vi "Teleop.vi"(0 "Call Context":T10) -> (6 "SubState 3":T4, 8 "SubState 4":T4, 9 "SubState 5":T9, 11 "Loop 3 Data":T5, 13 "Loop 4 Data":T3, 14 "SubState 0":T4=enum."driver control", 15 "Loop 1 Data":T7, 16 "Loop 0 Data":T8, 17 "SubState 1":T4, 18 "Loop 2 Data":T6, 19 "SubState 2":T4)   [LabVIEW 2013]
uses:
  typedefs/subStates.ctl
  <vilib>/Rock Robotics/WPI/DriverStation/WPI_DriverStationDerivedRobotMode.ctl
  typedefs/singleUseSubstate.ctl
  typedefs/Loop Datatypes/Loop 0 Datatype.ctl
  typedefs/Loop Datatypes/Loop 1 Datatype.ctl
  typedefs/Loop Datatypes/Loop 2 Datatype.ctl
  typedefs/Loop Datatypes/Loop 3 Datatype.ctl
  typedefs/Loop Datatypes/Loop 4 Datatype.ctl
  <vilib>/Rock Robotics/WPI/Joystick/WPI_JoystickDevRef.ctl
  <vilib>/Rock Robotics/WPI/Joystick/WPI_JoystickDeviceEnum.ctl
  typedefs/fg_typedef.ctl
  <vilib>/Rock Robotics/WPI/Joystick/WPI_JoystickGetSetRefNum.vi
panel:
  out "Drive to DC":bool
  out "JS2 Button 9":bool
  out "JS3":T1
  out "JS1":T1
  out "JS2":T1
  out "Exit Value":i32=-1
  # "Loop Data and Substates"
  # "Drive Loop"
  # "Shooter Pneumatics Loop"
  # "Pickup/Passing Belts Loop"
  # "Pickup Arm Loop"
  # "Unassigned Loop"
  # "Shifter Loop"
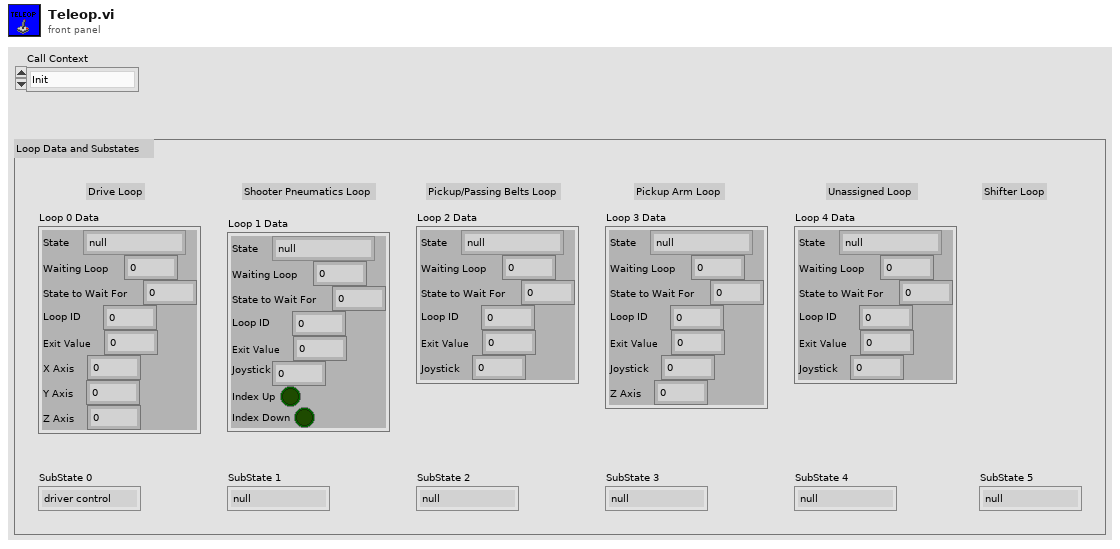
[diagram p1: front panel]
types:
  T1 = typedef "WPI_JoystickDevRef.ctl" = cluster{"Device":T2}
  T2 = typedef "WPI_JoystickDeviceEnum.ctl" = enum16{"USB 1", "USB 2", "USB 3", "USB 4", "Kinect 1", "Kinect 2"}
  T3 = typedef "Loop 4 Datatype.ctl" = cluster{"State":T4, "Waiting Loop":i32, "State to Wait For":i32, "Loop ID":i32, "Exit Value":i32, "Joystick":dbl}
  T4 = typedef "subStates.ctl" = enum16{"null", "wait", "driver control", "auto", "manual override", "hold position", "rotate", "pickup", "pass", "load", "cock", "goto shoot", "shoot", "end"}
  T5 = typedef "Loop 3 Datatype.ctl" = cluster{"State":T4, "Waiting Loop":i32, "State to Wait For":i32, "Loop ID":i32, "Exit Value":i32, "Joystick":dbl, "Z Axis":dbl}
  T6 = typedef "Loop 2 Datatype.ctl" = cluster{"State":T4, "Waiting Loop":i32, "State to Wait For":i32, "Loop ID":i32, "Exit Value":i32, "Joystick":dbl}
  T7 = typedef "Loop 1 Datatype.ctl" = cluster{"State":T4, "Waiting Loop":i32, "State to Wait For":i32, "Loop ID":i32, "Exit Value":i32, "Joystick":dbl, "Index Up":bool, "Index Down":bool}
  T8 = typedef "Loop 0 Datatype.ctl" = cluster{"State":T4, "Waiting Loop":i32, "State to Wait For":i32, "Loop ID":i32, "Exit Value":i32, "X Axis":dbl, "Y Axis":dbl, "Z Axis":dbl}
  T9 = typedef "singleUseSubstate.ctl" = enum16{"null", "wait", "shift high", "shift low"}
  T10 = typedef "WPI_DriverStationDerivedRobotMode.ctl" = enum16{"Init", "Execute", "Stop"}
  T11 = cluster{"axis 1 (x)":dbl, "axis 2 (y)":dbl, "axis 3 (throttle)":dbl, "axis 4":dbl, "axis 5":dbl, "axis 6":dbl}
  T12 = typedef "WPI_JoystickButtonState.ctl" = cluster{"Button 1":bool, "Button 2":bool, "Button 3":bool, "Button 4":bool, "Button 5":bool, "Button 6":bool, "Button 7":bool, "Button 8":bool, "Button 9":bool, "Button 10":bool, "Button 11":bool, "Button 12":bool}
  T13 = typedef "WPI_EncoderDevRef.ctl" = cluster{"DevStatus":errorcluster, "EncoderIndex":T14, "CounterIndex":T15, "DistancePerCount":dbl, "Decoding Type":T16}
  T14 = typedef "FPGA_EncoderIdx.ctl" = enum8{"Enc 0", "Enc 1", "Enc 2", "Enc 3", "Invalid"}
  T15 = typedef "FPGA_CounterCtrSystemIndex.ctl" = enum8{"Ctr 0", "Ctr 1", "Ctr 2", "Ctr 3", "Ctr 4", "Ctr 5", "Ctr 6", "Ctr 7", "Invalid"}
  T16 = typedef "WPI_EncoderType.ctl" = enum16{"1x", "2x", "4x"}
  T17 = typedef "fg_typedef.ctl" = enum16{"Get", "Set"}
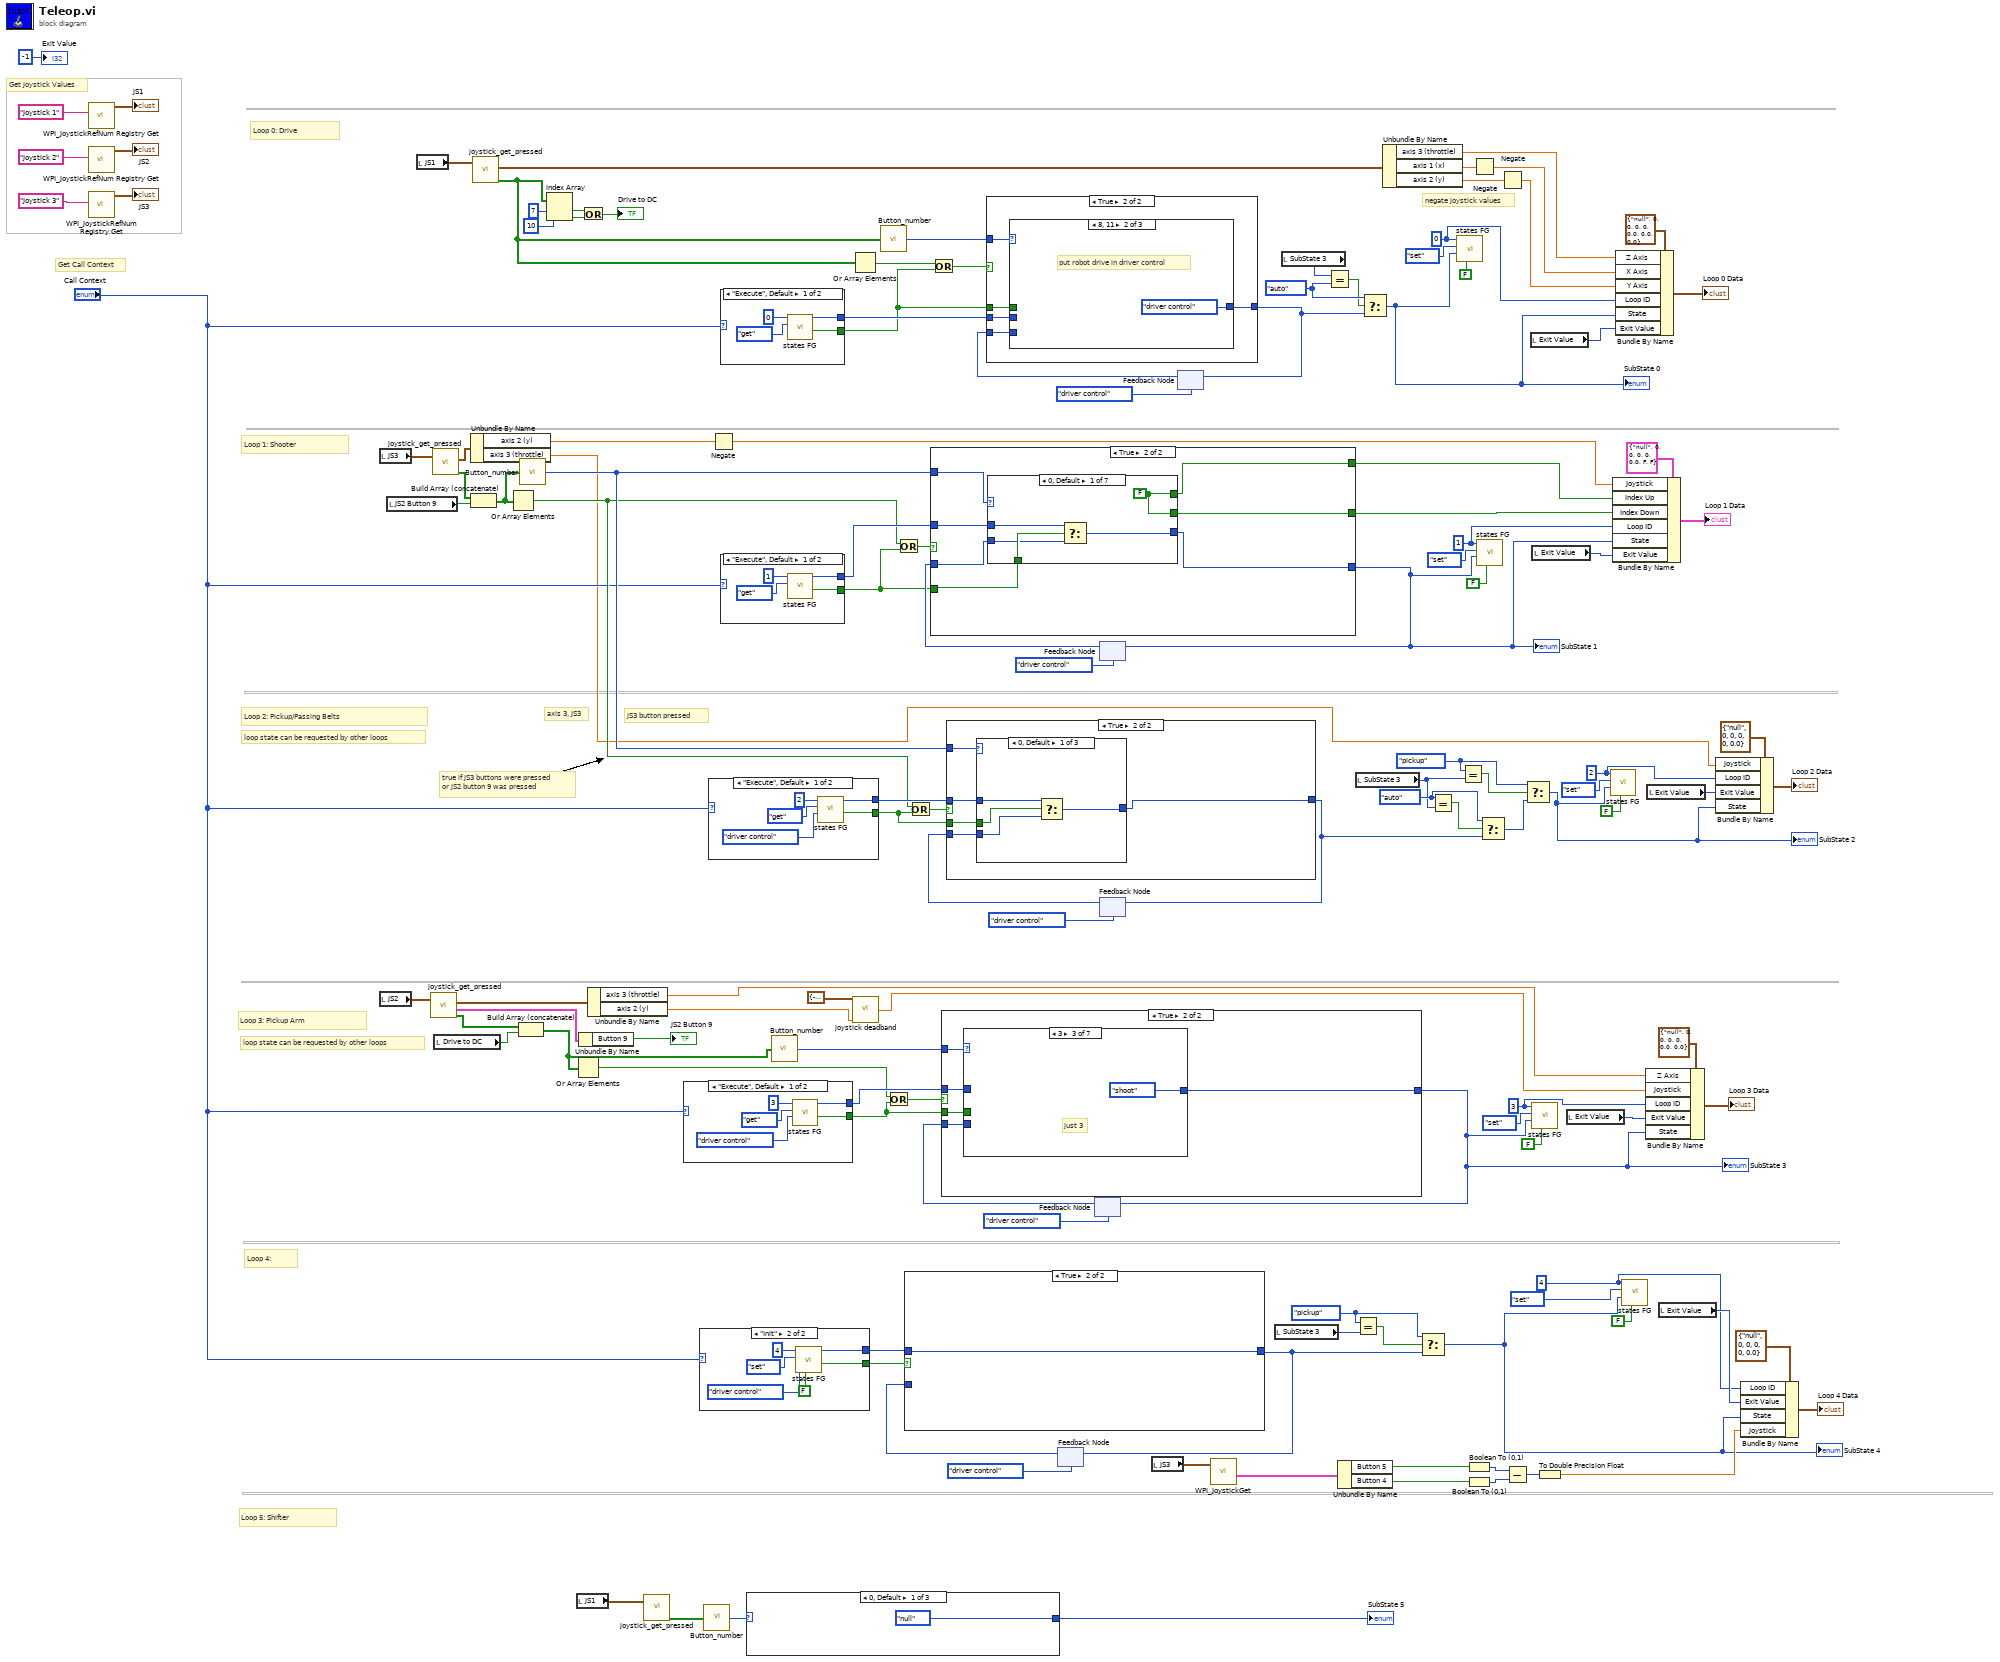
[diagram p0: block diagram]
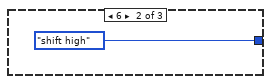
[diagram p2: hidden frame]
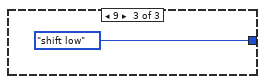
[diagram p3: hidden frame]
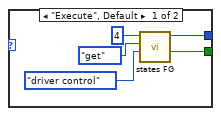
[diagram p5: hidden frame]
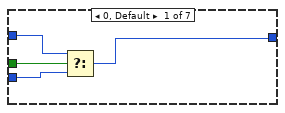
[diagram p7: hidden frame]
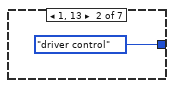
[diagram p8: hidden frame]
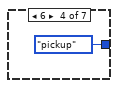
[diagram p9: hidden frame]
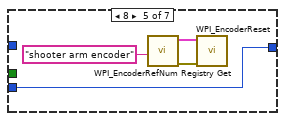
[diagram p10: hidden frame]
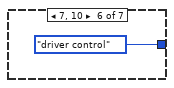
[diagram p11: hidden frame]
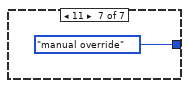
[diagram p12: hidden frame]
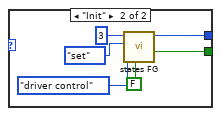
[diagram p13: hidden frame]
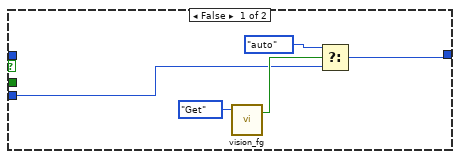
[diagram p14: hidden frame]
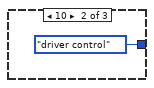
[diagram p15: hidden frame]
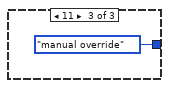
[diagram p16: hidden frame]
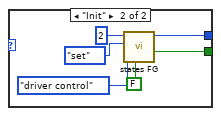
[diagram p17: hidden frame]
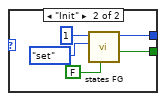
[diagram p18: hidden frame]
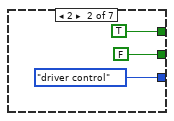
[diagram p20: hidden frame]
diagram:
  w26 = subStates."auto" ("y")
  w29 = subStates."auto" ("x")
  w36 = subStates."pickup" ("x")
  w38 = subStates."pickup" ("x")
  w91 = 4 ("Loop ID")
  w106 = 3 ("Loop ID")
  w107 = 2 ("Loop ID")
  w116 = 1 ("Loop ID")
  w118 = 0 ("Loop ID")
  # "true if JS3 buttons were pressed\nor JS2 button 9 was pressed"
  # "JS3 button pressed"
  # "axis 3, JS3"
  # "negate joystick values"
  # "Get Call Context"
  # "Get Joystick Values"
  # "Loop 4:"
  # "Loop 3: Pickup Arm"
  # "loop state can be requested by other loops"
  # "Loop 5: Shifter"
  # "Loop 2: Pickup/Passing Belts"
  # "Loop 1: Shooter"
  # "Loop 0: Drive"
  # "loop state can be requested by other loops"
  n1 = call <vilib>:"WPI_JoystickRefNum Registry Get.vi"("refnum name"="Joystick 1") -> ("JoystickDevRef"=→"JS1":T1)  [unwired: 9 in, 1 out]
  n2 = call <vilib>:"WPI_JoystickRefNum Registry Get.vi"("refnum name"="Joystick 2") -> ("JoystickDevRef"=→"JS2":T1)  [unwired: 9 in, 1 out]
  n3 = call <vilib>:"WPI_JoystickRefNum Registry Get.vi"("refnum name"="Joystick 3") -> ("JoystickDevRef"=→"JS3":T1)  [unwired: 9 in, 1 out]
  n4 = local read "JS3"() -> (w71:T1)
  n5 = local read "JS2"() -> (w49:T1)
  n6 = local read "JS2 Button 9"() -> (w56:bool)
  n7 = local read "JS1"() -> (w72:T1)
  n8 = call "joystick_get_pressed.vi"("JoystickDevRef 2"=w49) -> ("Axes"=w54:T11, "Buttons"=w8:T12, "Buttons Pressed?"=w52:bool[])  [unwired: 1 in, 1 out]
  n9 = call "joystick_get_pressed.vi"("JoystickDevRef 2"=w71) -> ("Axes"=w70:T11, "Buttons Pressed?"=w32:bool[])  [unwired: 1 in, 2 out]
  n10 = local read "Drive to DC"() -> (w11:bool)
  n11 = Unbundle By Name(w70) -> ("axis 2 (y)"=w79:dbl, "axis 3 (throttle)"=w6:dbl)
  n12 = Build Array (concatenate)(w32, w56) -> (w31:bool[])
  n13 = call "joystick_get_pressed.vi"("JoystickDevRef 2"=w72) -> ("Axes"=w78:T11, "Buttons Pressed?"=w17:bool[])  [unwired: 1 in, 2 out]
  n14 = Or Array Elements(Boolean array=w31) -> (logical OR=w59:bool)
  n15 = Build Array (concatenate)(w52, w11) -> (w5:bool[])
  n16 = call "Button_number.vi"("Button Array"=w31) -> ("Button Pressed"=w61:i32)
  n17 = Index Array(array=w17, index #1=7 ("index"), index #2=10 ("index")) -> (element #1=w14:bool, element #2=w13:bool)
  n18 = Or Array Elements(Boolean array=w5) -> (logical OR=w53:bool)
  n19 = local read "JS1"() -> (w1:T1)
  n20 = Unbundle By Name(w8) -> ("Button 9"=→"JS2 Button 9":bool)
  n21 = Or(x=w14, y=w13) -> (x .or. y?=→"Drive to DC":bool)
  n22 = Unbundle By Name(w54) -> ("axis 3 (throttle)"=w19:dbl, "axis 2 (y)"=w22:dbl)
  n23 = call "joystick_get_pressed.vi"("JoystickDevRef 2"=w1) -> ("Buttons Pressed?"=w3:bool[])  [unwired: 1 in, 3 out]
  n24 = case shown="\"Execute\", Default" "Call Context" {
    tunnel: [w137 w143] -> w50
    tunnel: [w135 w140] -> w104
    frame "Execute", Default {
      n25 = call "states FG.vi"("subState in"=subStates."driver control", "menu (get)"=enum16{"set", "get"}."get", "Loop ID"=3) -> ("exit out"=w137:bool, "subState out"=w135:T4)  [unwired: 5 in, 2 out]
    }
    frame "Init" {
      n26 = call "states FG.vi"("exit in"=FALSE, "subState in"=subStates."driver control", "menu (get)"=enum16{"set", "get"}."set", "Loop ID"=3) -> ("exit out"=w143:bool, "subState out"=w140:T4)  [unwired: 4 in, 2 out]
    }
  }
  n27 = case shown="\"Init\"" "Call Context" {
    tunnel: [w148 w154] -> w46
    tunnel: [w146 w151] -> w93
    frame "Execute", Default {
      n28 = call "states FG.vi"("subState in"=subStates."driver control", "menu (get)"=enum16{"set", "get"}."get", "Loop ID"=4) -> ("exit out"=w148:bool, "subState out"=w146:T4)  [unwired: 5 in, 2 out]
    }
    frame "Init" {
      n29 = call "states FG.vi"("exit in"=FALSE, "subState in"=subStates."driver control", "menu (get)"=enum16{"set", "get"}."set", "Loop ID"=4) -> ("exit out"=w154:bool, "subState out"=w151:T4)  [unwired: 4 in, 2 out]
    }
  }
  n30 = call "Button_number.vi"("Button Array"=w3) -> ("Button Pressed"=w2:i32)
  n31 = case shown="\"Execute\", Default" "Call Context" {
    tunnel: [w159 w165] -> w58
    tunnel: [w157 w162] -> w123
    frame "Execute", Default {
      n32 = call "states FG.vi"("subState in"=subStates."driver control", "menu (get)"=enum16{"set", "get"}."get", "Loop ID"=2) -> ("exit out"=w159:bool, "subState out"=w157:T4)  [unwired: 5 in, 2 out]
    }
    frame "Init" {
      n33 = call "states FG.vi"("exit in"=FALSE, "subState in"=subStates."driver control", "menu (get)"=enum16{"set", "get"}."set", "Loop ID"=2) -> ("exit out"=w165:bool, "subState out"=w162:T4)  [unwired: 4 in, 2 out]
    }
  }
  n34 = Negate(x=w79) -> (-x=w64:dbl)
  n35 = case shown="\"Execute\", Default" "Call Context" {
    tunnel: [w169 w174] -> w68
    tunnel: [w168 w172] -> w121
    frame "Execute", Default {
      n36 = call "states FG.vi"("menu (get)"=enum16{"set", "get"}."get", "Loop ID"=0) -> ("exit out"=w169:bool, "subState out"=w168:T4)  [unwired: 6 in, 2 out]
    }
    frame "Init" {
      n37 = call "states FG.vi"("exit in"=FALSE, "menu (get)"=enum16{"set", "get"}."set", "Loop ID"=0) -> ("exit out"=w174:bool, "subState out"=w172:T4)  [unwired: 5 in, 2 out]
    }
  }
  n38 = case shown="\"Execute\", Default" "Call Context" {
    tunnel: [w178 w183] -> w65
    tunnel: [w177 w181] -> w120
    frame "Execute", Default {
      n39 = call "states FG.vi"("menu (get)"=enum16{"set", "get"}."get", "Loop ID"=1) -> ("exit out"=w178:bool, "subState out"=w177:T4)  [unwired: 6 in, 2 out]
    }
    frame "Init" {
      n40 = call "states FG.vi"("exit in"=FALSE, "menu (get)"=enum16{"set", "get"}."set", "Loop ID"=1) -> ("exit out"=w183:bool, "subState out"=w181:T4)  [unwired: 5 in, 2 out]
    }
  }
  n41 = case shown="0, Default" w2 {
    tunnel: [singleUseSubstate."null" ("Enum") singleUseSubstate."shift high" ("Enum") singleUseSubstate."shift low" ("Enum")] -> w88
    frame 0, Default {
    }
    frame 6 {
    }
    frame 9 {
    }
  }
  "SubState 5" <- w88
  n42 = call "Button_number.vi"("Button Array"=w5) -> ("Button Pressed"=w51:i32)
  n43 = Or Array Elements(Boolean array=w17) -> (logical OR=w69:bool)
  n44 = call "joystick deadband.vi"("Joystick In"=w22, "Deadband Range"=cluster{"Deadband Min":dbl, "Deadband Max":dbl} {"Deadband Min"=-0.05, "Deadband Max"=0.05}) -> ("Joystick Out"=w4:dbl)  [unwired: 4 in]
  n45 = call "Button_number.vi"("Button Array"=w17) -> ("Button Pressed"=w77:i32)
  n46 = Or(x=w53, y=w50) -> (x .or. y?=w55:bool)
  n47 = Or(x=w59, y=w65) -> (x .or. y?=w66:bool)
  n48 = Or(x=w59, y=w58) -> (x .or. y?=w60:bool)
  n49 = Or(x=w69, y=w68) -> (x .or. y?=w67:bool)
  n50 = feedback #1(subStates."driver control" ("Drive SubState")) -> (w96:T4)
  n51 = case shown="True" w46 {
    tunnel: w96 -> [w189 _]
    tunnel: [w189 w190] -> w33
    tunnel: w93 -> [_ w190]
    frame False {
    }
    frame True {
    }
  }
  n52 = feedback-in #1(w33) -> ()
  n53 = feedback #2(subStates."driver control" ("Drive SubState")) -> (w101:T4)
  n54 = case shown="True" w55 {
    tunnel: w101 -> [w191 w192]
    tunnel: [w191 w193] -> w80
    tunnel: w104 -> [_ w194]
    tunnel: w51 -> [_ w196]
    tunnel: w50 -> [_ w195]
    frame False {
    }
    frame True {
      n55 = case shown="3" w196 {
        tunnel: w195 -> [w200 _ _ _ _ _ _]
        tunnel: w192 -> [w199 _ _ _ w204 _ _]
        tunnel: w194 -> [w198 _ _ _ _ _ _]
        tunnel: [w197 subStates."driver control" ("Drive SubState") subStates."shoot" ("Drive SubState") subStates."pickup" ("Drive SubState") w204 subStates."driver control" ("Drive SubState") subStates."manual override" ("Drive SubState")] -> w193
        frame 0, Default {
          n56 = Select(t=w198, s=w200, f=w199) -> (s? t:f=w197:T4)
        }
        frame 1, 13 {
        }
        frame 3 {
          # "just 3"
        }
        frame 6 {
        }
        frame 8 {
          n57 = call <vilib>:"WPI_EncoderRefNum Registry Get.vi"("refnum name"="shooter arm encoder") -> ("error out"=w206:errorcluster, "EncoderDevRef"=w205:T13)  [unwired: 9 in]
          n58 = call <vilib>:"WPI_EncoderReset.vi"("error in (no error)"=w206, "EncoderDevRef"=w205) -> ()  [unwired: 8 in, 2 out]
        }
        frame 7, 10 {
        }
        frame 11 {
        }
      }
    }
  }
  "SubState 3" <- w80
  n59 = feedback-in #2(w80) -> ()
  n60 = feedback #3(subStates."driver control" ("Drive SubState")) -> (w122:T4)
  n61 = case shown="True" w66 {
    tunnel: w122 -> [w210 w216]
    tunnel: [w210 w211] -> w81
    tunnel: w120 -> [_ w217]
    tunnel: w61 -> [_ w215]
    tunnel: w65 -> [_ w214]
    tunnel: [_ w213] -> w63
    tunnel: [_ w212] -> w62
    frame False {
      # "nothing pressed here, move along"
    }
    frame True {
      n62 = case shown="0, Default" w215 {
        tunnel: w217 -> [w221 _ _ _ _ _ _]
        tunnel: w216 -> [w220 _ _ _ _ _ w239]
        tunnel: [w219 subStates."driver control" ("Drive SubState") subStates."driver control" ("Drive SubState") subStates."driver control" ("Drive SubState") subStates."manual override" ("Drive SubState") subStates."driver control" ("Drive SubState") w239] -> w211
        tunnel: w214 -> [w222 _ _ _ _ _ _]
        tunnel: [w218 TRUE FALSE w229 w231 w233 w235] -> w213
        tunnel: [w218 FALSE TRUE w229 w231 w233 w235] -> w212
        frame 0, Default {
          w218 = FALSE
          n63 = Select(t=w221, s=w222, f=w220) -> (s? t:f=w219:T4)
        }
        frame 2 {
        }
        frame 3 {
        }
        frame 6 {
          w229 = FALSE
        }
        frame 9 {
          w231 = FALSE
        }
        frame 8, 10 {
          w233 = FALSE
        }
        frame 13 {
          w235 = FALSE
          n64 = call <vilib>:"WPI_EncoderRefNum Registry Get.vi"("refnum name"="auger encoder") -> ("error out"=w237:errorcluster, "EncoderDevRef"=w236:T13)  [unwired: 9 in]
          n65 = call <vilib>:"WPI_EncoderReset.vi"("error in (no error)"=w237, "EncoderDevRef"=w236) -> ()  [unwired: 8 in, 2 out]
        }
      }
    }
  }
  "SubState 1" <- w81
  n66 = feedback-in #3(w81) -> ()
  n67 = feedback #4(subStates."driver control" ("Drive SubState")) -> (w126:T4)
  n68 = case shown="True" w60 {
    tunnel: w126 -> [w240 w246]
    tunnel: [w241 w245] -> w9
    tunnel: w123 -> [_ w247]
    tunnel: w61 -> [_ w249]
    tunnel: w58 -> [_ w248]
    frame False {
      n69 = call "vision_fg.vi"("Menu"=fg_typedef."Get") -> ("Enabled?"=w243:bool)  [unwired: 2 in, 1 out]
      n70 = Select(t=subStates."auto", s=w243, f=w240) -> (s? t:f=w241:T4)
    }
    frame True {
      n71 = case shown="0, Default" w249 {
        tunnel: w248 -> [w253 _ _]
        tunnel: w247 -> [w252 _ _]
        tunnel: w246 -> [w251 _ _]
        tunnel: [w250 subStates."driver control" ("Drive SubState") subStates."manual override" ("Drive SubState")] -> w245
        frame 0, Default {
          n72 = Select(t=w252, s=w253, f=w251) -> (s? t:f=w250:T4)
        }
        frame 10 {
        }
        frame 11 {
        }
      }
    }
  }
  n73 = feedback-in #4(w9) -> ()
  n74 = local read "JS3"() -> (w48:T1)
  n75 = feedback #5(subStates."driver control" ("Drive SubState")) -> (w128:T4)
  n76 = case shown="True" w67 {
    tunnel: w128 -> [w256 w258]
    tunnel: [w256 w257] -> w20
    tunnel: w121 -> [_ w259]
    tunnel: w77 -> [_ w261]
    tunnel: w68 -> [_ w260]
    frame False {
      # "keep current state, no change necessary"
    }
    frame True {
      n77 = case shown="8, 11" w261 {
        tunnel: w260 -> [w265 _ _]
        tunnel: w259 -> [w264 _ _]
        tunnel: w258 -> [w263 _ w271]
        tunnel: [w262 subStates."driver control" ("Drive SubState") w267] -> w257
        frame 0, Default {
          n78 = Select(t=w264, s=w265, f=w263) -> (s? t:f=w262:T4)
        }
        frame 8, 11 {
          # "put robot drive in driver control"
        }
        frame 7 {
          w268 = subStates."hold position" ("x")
          # "button 7, hold position toggle"
          n79 = Equal?(x=w268, y=w271) -> (x = y?=w270:bool)
          n80 = Select(t=subStates."driver control" ("Drive SubState"), s=w270, f=w268) -> (s? t:f=w267:T4)
        }
      }
    }
  }
  n81 = feedback-in #5(w20) -> ()
  n82 = call <vilib>:"WPI_JoystickGet.vi"("JoystickDevRef"=w48) -> ("Buttons"=w47:T12)  [unwired: 4 in, 2 out]
  n83 = local read "SubState 3"() -> (w35:T4)
  n84 = local read "SubState 3"() -> (w24:T4)
  n85 = Equal?(x=w24, y=w26) -> (x = y?=w25:bool)
  n86 = Unbundle By Name(w47) -> ("Button 5"=w45:bool, "Button 4"=w44:bool)
  n87 = local read "SubState 3"() -> (w27:T4)
  n88 = Equal?(x=w36, y=w35) -> (x = y?=w37:bool)
  n89 = Select(t=w26, s=w25, f=w20) -> (s? t:f=w23:T4)
  "SubState 0" <- w23
  n90 = Unbundle By Name(w78) -> ("axis 3 (throttle)"=w18:dbl, "axis 1 (x)"=w85:dbl, "axis 2 (y)"=w84:dbl)
  n91 = Select(t=w36, s=w37, f=w33) -> (s? t:f=w34:T4)
  "SubState 4" <- w34
  n92 = Equal?(x=w29, y=w27) -> (x = y?=w30:bool)
  n93 = call "states FG.vi"("exit in"=FALSE, "subState in"=w23, "menu (get)"=enum16{"set", "get"}."set", "Loop ID"=w118) -> ()  [unwired: 4 in, 4 out]
  n94 = Equal?(x=w38, y=w27) -> (x = y?=w39:bool)
  n95 = Boolean To (0,1)(Boolean=w45) -> (0, 1=w42:i16)
  n96 = Boolean To (0,1)(Boolean=w44) -> (0, 1=w43:i16)
  n97 = Negate(x=w85) -> (-x=w83:dbl)
  n98 = call "states FG.vi"("exit in"=FALSE, "subState in"=w81, "menu (get)"=enum16{"set", "get"}."set", "Loop ID"=w116) -> ()  [unwired: 4 in, 4 out]
  n99 = Select(t=w29, s=w30, f=w9) -> (s? t:f=w28:T4)
  n100 = Negate(x=w84) -> (-x=w82:dbl)
  n101 = Subtract(x=w42, y=w43) -> (x-y=w41:i16)
  n102 = Select(t=w38, s=w39, f=w28) -> (s? t:f=w10:T4)
  "SubState 2" <- w10
  n103 = local read "Exit Value"() -> (w114:i32)
  n104 = local read "Exit Value"() -> (w113:i32)
  n105 = call "states FG.vi"("exit in"=FALSE, "subState in"=w80, "menu (get)"=enum16{"set", "get"}."set", "Loop ID"=w106) -> ()  [unwired: 4 in, 4 out]
  n106 = To Double Precision Float(number=w41) -> (double precision float=w40:dbl)
  n107 = local read "Exit Value"() -> (w105:i32)
  n108 = call "states FG.vi"("exit in"=FALSE, "subState in"=w10, "menu (get)"=enum16{"set", "get"}."set", "Loop ID"=w107) -> ()  [unwired: 4 in, 4 out]
  n109 = Bundle By Name(cluster=T7 {"State"=enum."null", "Waiting Loop"=0, "State to Wait For"=0, "Loop ID"=0, "Exit Value"=0, "Joystick"=0.0, "Index Up"=FALSE, "Index Down"=FALSE} ("Cluster"), "Joystick"=w64, "Index Up"=w63, "Index Down"=w62, "Loop ID"=w116, "State"=w81, "Exit Value"=w113) -> (→"Loop 1 Data":T7)
  n110 = Bundle By Name(cluster=T8 {"State"=enum."null", "Waiting Loop"=0, "State to Wait For"=0, "Loop ID"=0, "Exit Value"=0, "X Axis"=0.0, "Y Axis"=0.0, "Z Axis"=0.0} ("Cluster"), "Z Axis"=w18, "X Axis"=w83, "Y Axis"=w82, "Loop ID"=w118, "State"=w23, "Exit Value"=w114) -> (→"Loop 0 Data":T8)
  n111 = call "states FG.vi"("exit in"=FALSE, "subState in"=w34, "menu (get)"=enum16{"set", "get"}."set", "Loop ID"=w91) -> ()  [unwired: 4 in, 4 out]
  n112 = Bundle By Name(cluster=T5 {"State"=enum."null", "Waiting Loop"=0, "State to Wait For"=0, "Loop ID"=0, "Exit Value"=0, "Joystick"=0.0, "Z Axis"=0.0} ("Loop 3 Data"), "Z Axis"=w19, "Joystick"=w4, "Loop ID"=w106, "Exit Value"=w105, "State"=w80) -> (→"Loop 3 Data":T5)
  n113 = local read "Exit Value"() -> (w108:i32)
  n114 = local read "Exit Value"() -> (w92:i32)
  n115 = Bundle By Name(cluster=T6 {"State"=enum."null", "Waiting Loop"=0, "State to Wait For"=0, "Loop ID"=0, "Exit Value"=0, "Joystick"=0.0} ("Loop 2 Data"), "Joystick"=w6, "Loop ID"=w107, "Exit Value"=w108, "State"=w10) -> (→"Loop 2 Data":T6)
  n116 = Bundle By Name(cluster=T3 {"State"=enum."null", "Waiting Loop"=0, "State to Wait For"=0, "Loop ID"=0, "Exit Value"=0, "Joystick"=0.0} ("Loop 4 Data"), "Loop ID"=w91, "Exit Value"=w92, "State"=w34, "Joystick"=w40) -> (→"Loop 4 Data":T3)
  "Exit Value" <- -1 ("Exit Value")
